vi "Get Value (String Value).vi"(8 "error in (no error)":errorcluster, 10 "key":string, 11 "JSON Value in":refnum<class "JSON Value.lvclass">) -> (0 "error out":errorcluster, 2 "value":string)   [LabVIEW 2016, in "JSON Value.lvclass"]
uses:
  JSON Value.lvclass
  Read Value/Read value as String.vi
  Get Value (JSON).vi
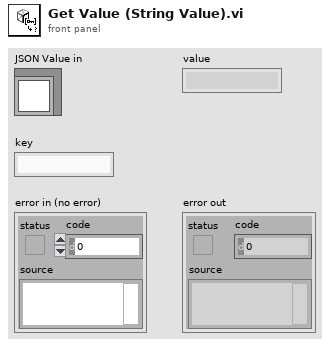
[diagram p1: front panel]
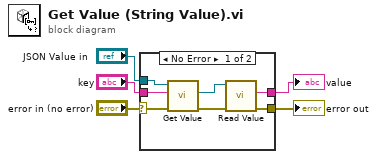
[diagram p0: block diagram]
diagram:
  n1 = case shown="No Error" "error in (no error)" {
    selector: "error in (no error)" -> [w10 w13]
    tunnel: [w9 w13] -> w4
    tunnel: "JSON Value in" -> [w12 _]
    tunnel: "key" -> [w11 _]
    tunnel: [w6 _] -> w1
    frame No Error {
      n2 = call-poly "Get Value.vi"("error in (no error)"=w10, "key"=w11, "JSON Value in"=w12) -> ("error out"=w8:errorcluster, "JSON Value out"=w7:refnum<class "JSON Value.lvclass">)  [unwired: 7 in]
      n3 = call-poly "Read Value.vi"("error in (no error)"=w8, "JSON String in"=w7) -> ("error out"=w9:errorcluster, "value"=w6:string)  [unwired: 8 in]
    }
    frame Error {
    }
  }
  "error out" <- w4
  "value" <- w1
